vi "libssh2_channel_forward_accept.vi"(8 "error in (no error)":errorcluster, 11 "listener":u64) -> (0 "error out":errorcluster, 3 "return value":u64)   [LabVIEW 2013, in "libssh2.lvlib"]
uses:
  libssh2.lvlib
  libssh2.dll
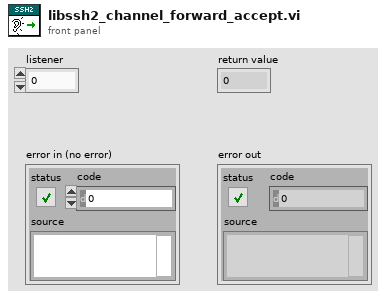
[diagram p1: front panel]
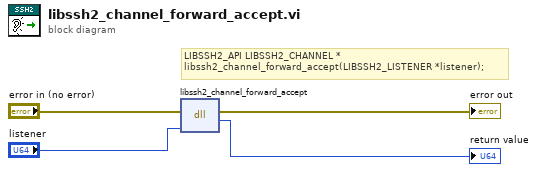
[diagram p0: block diagram]
diagram:
  # "LIBSSH2_API LIBSSH2_CHANNEL *\nlibssh2_channel_forward_accept(LIBSSH2_LISTENER *listener);"
  n1 = dll-call lib="C:/Users/pasca/source/repos/libssh2-labview/libssh2**.*" fn="libssh2_channel_forward_accept"(error in="error in (no error)", "listener"="listener") -> (error out=→"error out":errorcluster, "return value"=→"return value":u64)  [unwired: 3 in, 1 out]
